vi "Get Batch Controls.vi"(8 "error in (no error)":errorcluster, 10 "Control Names":string[](array[string]), 11 "Controls_Mgr in":refnum<class "Controls_Mgr.lvclass">) -> (0 "error out":errorcluster, 2 "Values":variant[](array[variant]), 3 "Controls_Mgr out":refnum<class "Controls_Mgr.lvclass">)   [LabVIEW 2015, in "Generic Module Library.lvlib" / "Template G_Module.lvlib" / "Controls_Mgr.lvclass"]
uses:
  Controls_Mgr.lvclass
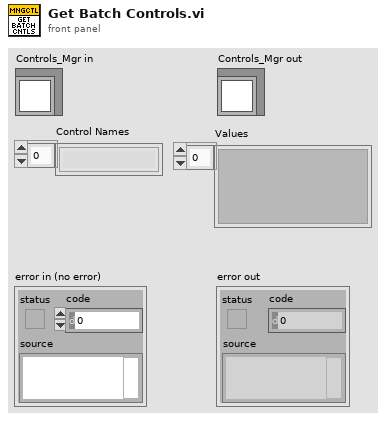
[diagram p1: front panel]
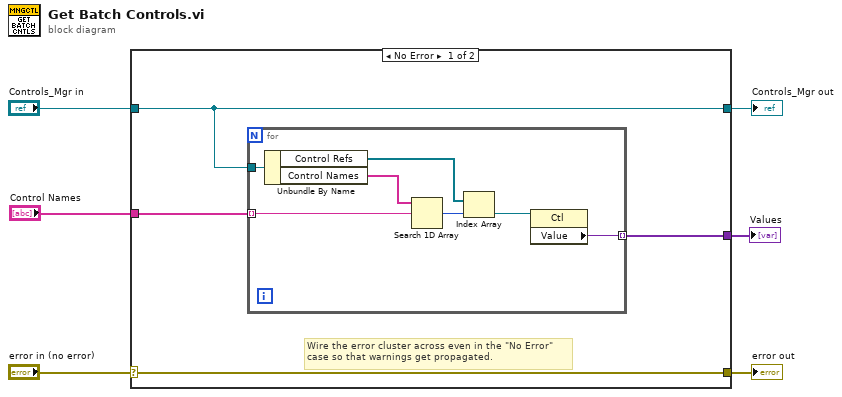
[diagram p0: block diagram]
diagram:
  n1 = case shown="No Error" "error in (no error)" {
    selector: "error in (no error)" -> [w10 w19]
    tunnel: [w10 w19] -> w5
    tunnel: [w9 w18] -> w4
    tunnel: "Controls_Mgr in" -> [w9 w18]
    tunnel: "Control Names" -> [w8 _]
    tunnel: [w7 _] -> w1
    frame No Error {
      # "Wire the error cluster across even in the \"No Error\"\ncase so that warnings get propagated."
      n2 = for {
        tunnel: w9 -> [w17]
        tunnel: w8 -> [w13] mode=indexing
        tunnel: [w11] -> w7 mode=indexing
        n3 = Unbundle By Name(w17) -> ("Control Refs"=w15:refnum<vi>[], "Control Names"=w14:string[])
        n4 = Search 1D Array(1D array=w14, element=w13) -> (index of element=w16:i32)  [unwired: 1 in]
        n5 = Index Array(array=w15, index=w16) -> (element=w12:refnum<vi>)
        n6 = property class="Ctl"(reference=w12) -> ("Value"=w11:variant)  [unwired: 1 in, 2 out]
      }
    }
    frame Error {
    }
  }
  "error out" <- w5
  "Controls_Mgr out" <- w4
  "Values" <- w1
